vi "DataFinder PreProcess Results.vi"(9 "Raw Results (empty)":string[][](array[string]), 11 "RUNSELECT (\"\")":string) -> (0 "Results":string[][](array[string]), 1 "Items":string[][](array[string]), 2 "Item Filepaths":string[](array[string]), 3 "Item Filenames":string[](array[string]), 6 "runs":T1[](array[typedef]))   [LabVIEW 2011]
uses:
  www/cgi-bin/_cgi-lib/TDM_INDEX Record.ctl
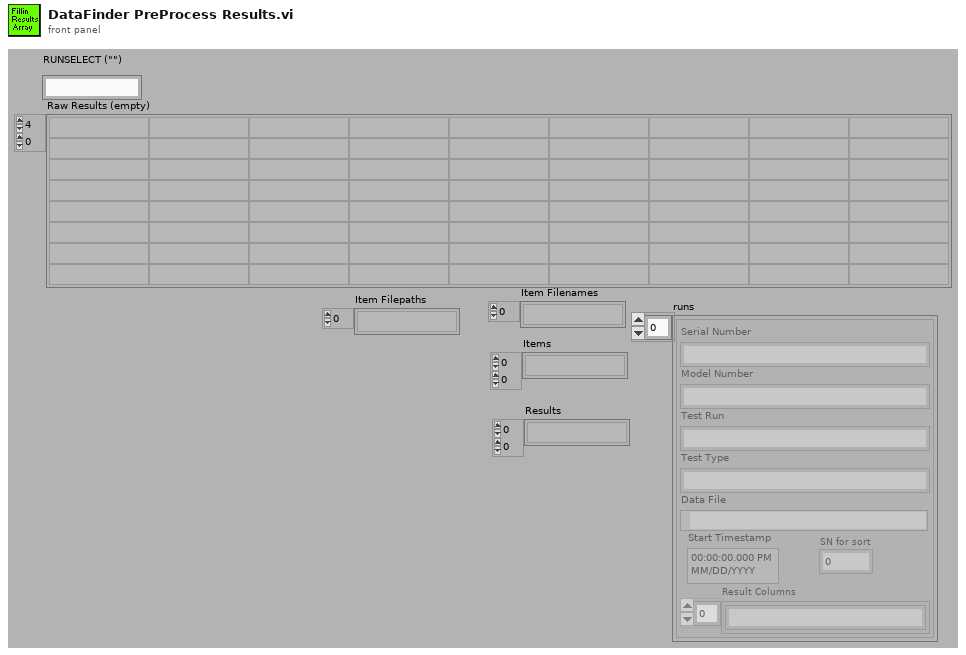
[diagram p1: front panel]
types:
  T1 = typedef "TDM_INDEX Record.ctl" = cluster{"Model Number":string, "SN for sort":i32, "Test Type":string, "Test Run":string, "Serial Number":string, "Start Timestamp":timestamp, "Data File":path, "Result Columns":string[]}
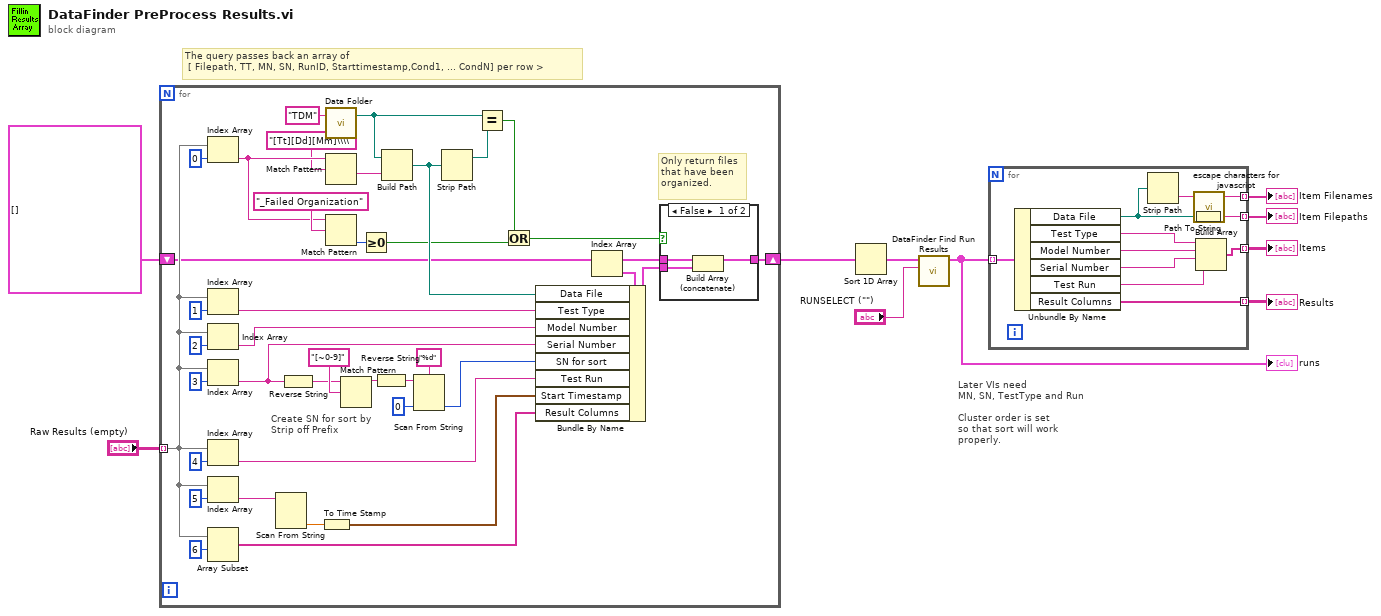
[diagram p0: block diagram]
diagram:
  # "The query passes back an array of\n [ Filepath, TT, MN, SN, RunID, Starttimestamp,Cond1, ... CondN] per row >"
  # "Later VIs need \nMN, SN, TestType and Run\n\nCluster order is set\nso that sort will work\nproperly."
  n1 = for {
    tunnel: "Raw Results (empty)" -> [w36] mode=indexing
    shift-right: [w26] -> w1
    shift-left: T1[] [] ("array") -> [w15]
    # "Only return files\nthat have been \norganized."
    # "Create SN for sort by\nStrip off Prefix"
    n2 = Index Array(array=w36, index=0) -> (element=w21:string)
    n3 = Index Array(array=w36, index=1) -> (element=w47:string)
    n4 = Index Array(array=w36, index=2) -> (element=w38:string)
    n5 = Index Array(array=w36, index=3) -> (element=w28:string)
    n6 = Index Array(array=w36, index=4) -> (element=w37:string)
    n7 = Index Array(array=w36, index=5) -> (element=w39:string)
    n8 = Array Subset(array=w36, index=6) -> (w35:string[])  [unwired: 1 in]
    n9 = Scan From String(input string=w39) -> (output 1=w43:dbl)  [unwired: 3 in, 4 out]
    n10 = Reverse String(1:w28) -> (0:w31:string)
    n11 = To Time Stamp(1:w43) -> (0:w42:timestamp)
    n12 = call "Data Folder.vi"("Relative Path (\"\" - Folder)"="TDM" ("Relative Path (\"\" - Folder)")) -> ("Data Folder"=w18:path)  [unwired: 2 in]
    n13 = Match Pattern(string=w21, regular expression="[Tt][Dd][Mm]\\\\") -> (after substring=w19:string)  [unwired: 1 in, 3 out]
    n14 = Match Pattern(string=w21, regular expression="_Failed Organization") -> (offset past match=w23:i32)  [unwired: 1 in, 3 out]
    n15 = Match Pattern(string=w31, regular expression="[~0-9]" ("format string")) -> (before substring=w29:string)  [unwired: 4 out]
    n16 = Greater Or Equal To 0?(x=w23) -> (x >= 0?=w12:bool)
    n17 = Reverse String(1:w29) -> (0:w30:string)
    n18 = Build Path(base path=w18, name or relative path=w19) -> (appended path=w17:path)
    n19 = Scan From String(format string="%d", input string=w30, default 1=0 ("default value 1")) -> (output 1=w11:i32)  [unwired: 2 in, 3 out]
    n20 = Strip Path(path=w17) -> (stripped path=w16:path)  [unwired: 1 out]
    n21 = Equal?(x=w18, y=w16) -> (x = y?=w13:bool)
    n22 = Or(x=w13, y=w12) -> (x .or. y?=w22:bool)
    n23 = Index Array(array=w15) -> (element=w14:T1)  [unwired: 1 in]
    n24 = Bundle By Name(cluster=w14, "Data File"=w17, "Test Type"=w47, "Model Number"=w38, "Serial Number"=w28, "SN for sort"=w11, "Test Run"=w37, "Start Timestamp"=w42, "Result Columns"=w35) -> (w25:T1)
    n25 = case shown="False" w22 {
      tunnel: w15 -> [w52 w53]
      tunnel: [w51 w53] -> w26
      tunnel: w25 -> [w50 _]
      frame False {
        n26 = Build Array (concatenate)(w52, w50) -> (w51:T1[])
      }
      frame True {
      }
    }
  }
  n27 = Sort 1D Array(array=w1) -> (sorted array=w9:T1[])
  n28 = call "DataFinder Find Run Results.vi"("RUNSELECT (Most Recent, First, ALL)"="RUNSELECT (\"\")", "Run Results (empty)"=w9) -> ("Filtered Run Results"=w7:T1[])  [unwired: 9 out]
  "runs" <- w7
  n29 = for {
    tunnel: w7 -> [w64] mode=indexing
    tunnel: [w63] -> w6 mode=indexing
    tunnel: [w58] -> w5 mode=indexing
    tunnel: [w56] -> w4 mode=indexing
    tunnel: [w54] -> w3 mode=indexing
    n30 = Unbundle By Name(w64) -> ("Data File"=w55:path, "Test Type"=w62:string, "Model Number"=w61:string, "Serial Number"=w60:string, "Test Run"=w59:string, "Result Columns"=w63:string[])
    n31 = Strip Path(path=w55) -> (name=w57:string)  [unwired: 1 out]
    n32 = Path To String(path=w55) -> (string=w54:string)
    n33 = call "escape characters for javascript.vi"("String (\"\")"=w57) -> ("escaped String"=w56:string)  [unwired: 4 out]
    n34 = Build Array(w62, w61, w60, w59) -> (w58:string[])
  }
  "Results" <- w6
  "Items" <- w5
  "Item Filenames" <- w4
  "Item Filepaths" <- w3
